vi "PID Test.vi"(9 "Straigtness Bias":dbl(slide)=-0.016713091922005565 scale=10.0..100.0, 10 "global bearing":dbl, 11 "Speed":dbl(slide)=-0.016713091922005565 scale=-10.0..10.0) -> ()   [LabVIEW 2017]
uses:
  <vilib>/myRIO/Instrument Drivers/Utilities/Utilities.lvlib
panel:
  out "rad/s":dbl
  out "dx/dt":dbl
  out "Waveform Chart":T1(graph)
  in  "milliseconds to wait":u32=100
  in  "stop":bool
  in  "PID gains":T2={"proportional gain (Kc)"=0.015, "integral time (Ti, min)"=0.003, "derivative time (Td, min)"=0.0} {"derivative time (Td, min)" format="%.6f"; "integral time (Ti, min)" format="%.6f"; "proportional gain (Kc)" format="%.6f"}
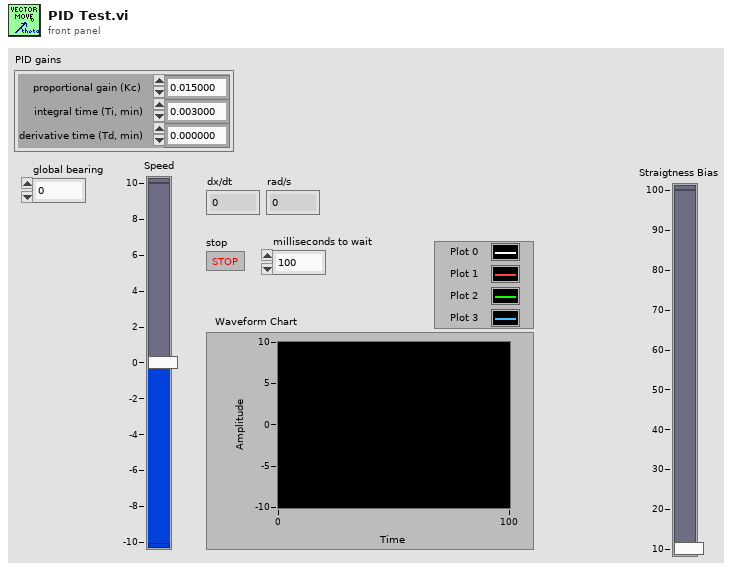
[diagram p1: front panel]
types:
  T1 = cluster{"Setpoint":dbl, "Setpoint":dbl, "dx/dt":dbl, "dx/dt":dbl}
  T2 = cluster{"proportional gain (Kc)":dbl, "integral time (Ti, min)":dbl, "derivative time (Td, min)":dbl}
  T3 = cluster{"Setpoint":dbl, "output":dbl, "dx/dt":dbl}
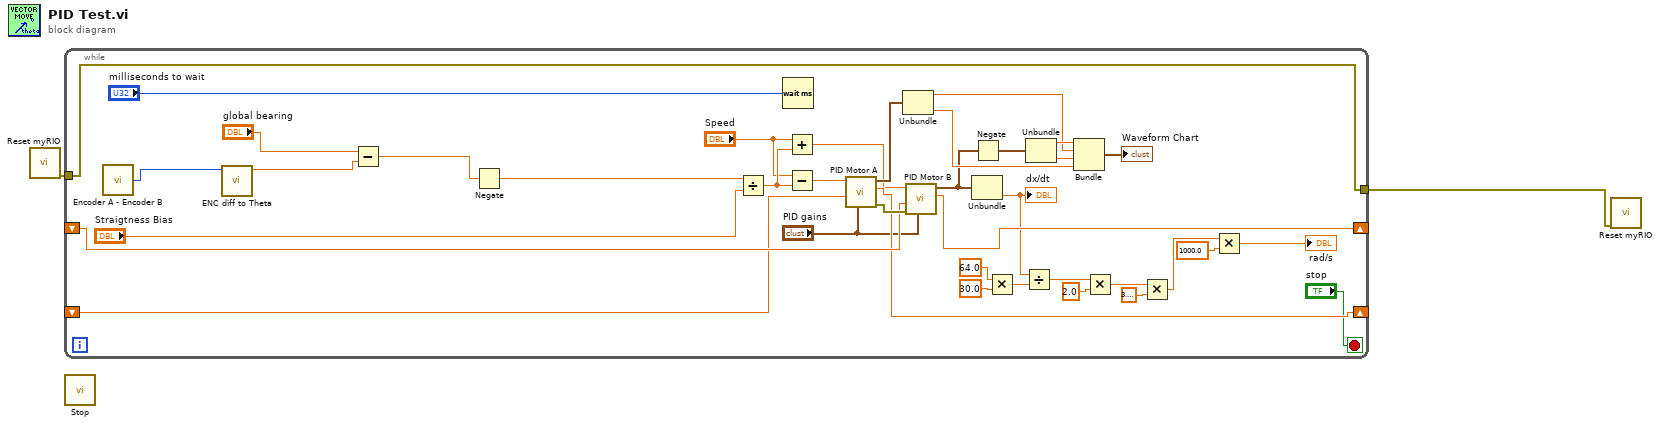
[diagram p0: block diagram]
diagram:
  n1 = call <vilib>:"Reset myRIO.vi"() -> ("error out"=w1:errorcluster)  [unwired: 11 in]
  n2 = while {
    shift-right: [w39] -> _
    shift-left: _ -> [w38]
    shift-right: [w37] -> _
    shift-left: _ -> [w36]
    tunnel: [w13] -> w2
    tunnel: w1 -> [w13]
    stop <- "stop" stop-if-true
    n3 = call "Encoder A - Encoder B.vi"() -> ("x-y"=w7:i32)  [unwired: 1 in]
    n4 = call "ENC diff to Theta.vi"("ENC  A - B"=w7) -> ("theta"=w5:dbl)  [unwired: 9 in, 1 out]
    n5 = Subtract(x="global bearing", y=w5) -> (x-y=w4:dbl)
    n6 = Negate(x=w4) -> (-x=w3:dbl)
    n7 = Divide(x=w3, y="Straigtness Bias") -> (x/y=w10:dbl)
    n8 = Wait (ms)(milliseconds to wait="milliseconds to wait") -> ()  [unwired: 1 out]
    n9 = Add(x="Speed", y=w10) -> (x+y=w11:dbl)
    n10 = Subtract(x="Speed", y=w10) -> (x-y=w12:dbl)
    n11 = call "PID Motor A.vi"("PID gains"="PID gains", "input"=w36, "Setpoint A0"=w12) -> ("error out"=w40:errorcluster, "output"=w37:dbl, "Speed A0"=w31:T3)  [unwired: 3 in, 3 out]
    n12 = Unbundle(w31) -> ("Setpoint"=w29:dbl, "dx/dt"=w27:dbl)  [unwired: 1 out]
    n13 = call "PID Motor B.vi"("PID gains"="PID gains", "error in (no error)"=w40, "input"=w38, "Setpoint B0"=w11) -> ("output"=w39:dbl, "Speed B0"=w25:T3)  [unwired: 2 in, 4 out]
    n14 = Unbundle(w25) -> ("dx/dt"=w21:dbl)  [unwired: 2 out]
    "dx/dt" <- w21
    n15 = Negate(x=w25) -> (-x=w32:T3)
    n16 = Multiply(x=64.0 ("y"), y=30.0) -> (x*y=w23:dbl)
    n17 = Divide(x=w21, y=w23) -> (x/y=w17:dbl)
    n18 = Unbundle(w32) -> ("Setpoint"=w30:dbl, "dx/dt"=w28:dbl)  [unwired: 1 out]
    n19 = Bundle("Setpoint"=w30, "Setpoint"=w29, "dx/dt"=w28, "dx/dt"=w27) -> (→"Waveform Chart":T1)  [unwired: 1 in]
    n20 = Multiply(x=w17, y=2.0) -> (x*y=w18:dbl)
    n21 = Multiply(x=w18, y=3.141592653589793) -> (x*y=w15:dbl)
    n22 = Multiply(x=w15, y=1000.0) -> (x*y=→"rad/s":dbl)
  }
  n23 = call "Stop.vi"() -> ()  [unwired: 10 in, 2 out]
  n24 = call <vilib>:"Reset myRIO.vi"("error in (no error)"=w2) -> ()  [unwired: 10 in, 1 out]
